vi "Update.vi"(9 "Player 2 Position":refnum<class "Vector 2D.lvclass">, 10 "Player 1 Position":refnum<class "Vector 2D.lvclass">, 11 "Camera in":refnum<class "Camera.lvclass">) -> (3 "Camera out":refnum<class "Camera.lvclass">)   [LabVIEW 2021, in "Camera.lvclass"]
uses:
  Camera.lvclass
  Re-use Libraries/Vector 2D/Vector 2D.lvclass
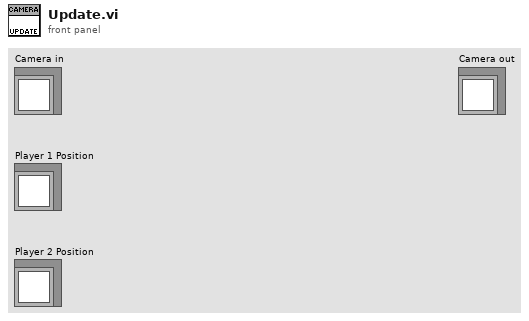
[diagram p1: front panel]
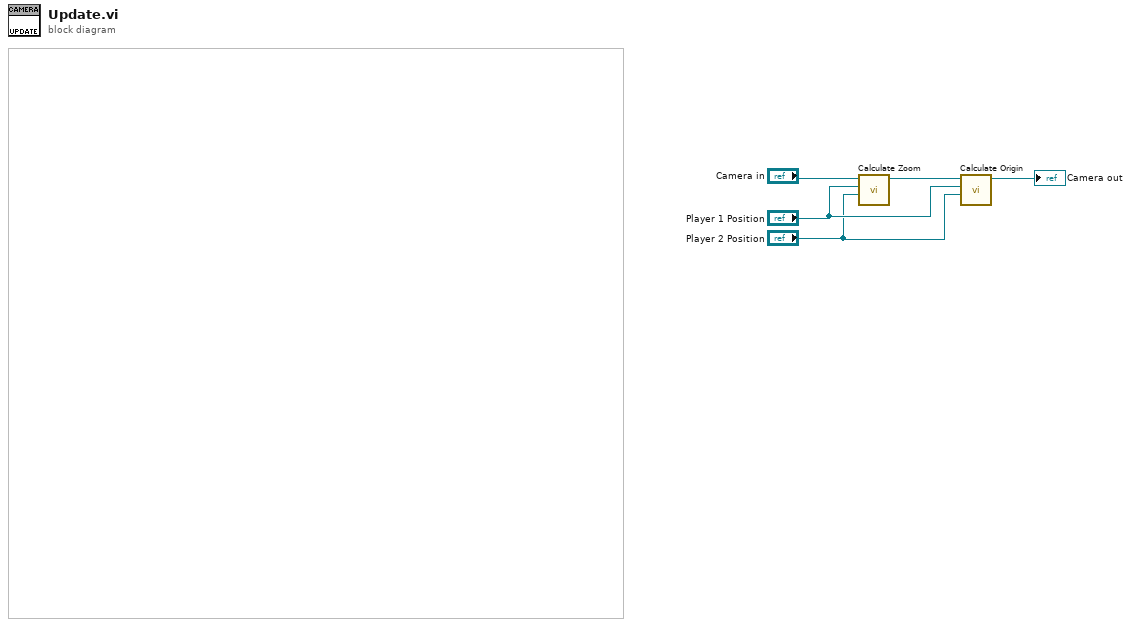
[diagram p0: block diagram]
diagram:
  n1 = call "Calculate Zoom.vi"("Player 2 Position"="Player 2 Position", "Player 1 Position"="Player 1 Position", "Camera in"="Camera in") -> ("Camera out"=w1:refnum<class "Camera.lvclass">)  [unwired: 8 in]
  n2 = call "Calculate Origin.vi"("Player 2 Position"="Player 2 Position", "Player 1 Position"="Player 1 Position", "Camera in"=w1) -> ("Camera out"=→"Camera out":refnum<class "Camera.lvclass">)  [unwired: 8 in]
